vi "ExTestPutRowI32.vi"() -> ()   [LabVIEW 2010]
panel:
  out "Image Display 2":i32[][](graph)
  out "error out":errorcluster
  in  "error in (no error)":errorcluster
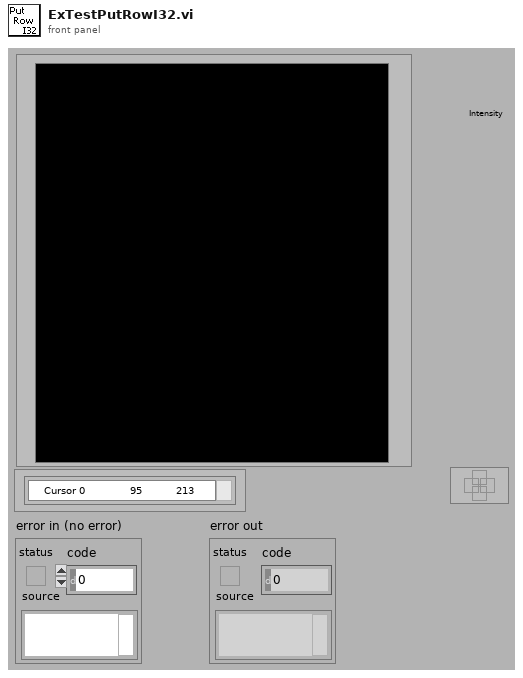
[diagram p1: front panel]
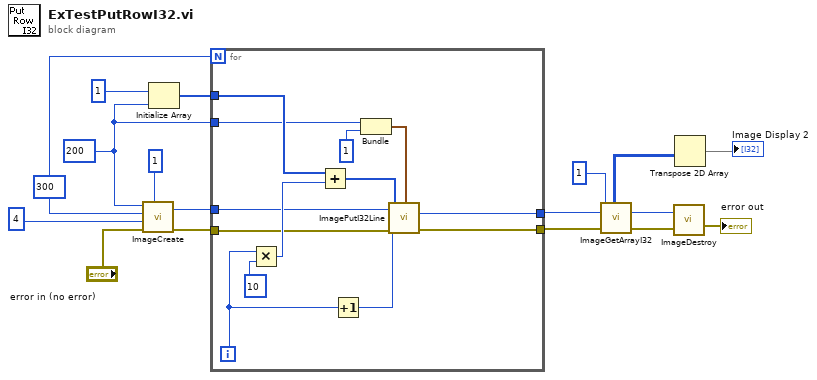
[diagram p0: block diagram]
diagram:
  w6 = 200
  w15 = 300
  n1 = call <userlib>:"ImageCreate.vi"("X dimension"=w6, "Y dimension"=w15, "Data Type"=4, "error in"="error in (no error)", "Number Of Frames"=1) -> ("Image Handle"=w7:u32, "error out"=w9:errorcluster)
  n2 = Initialize Array(1, w6) -> (w8:i32[])
  n3 = for {
    N: w15 -> [_]
    tunnel: w9 -> [w24]
    tunnel: w8 -> [w27]
    tunnel: w7 -> [w23]
    tunnel: w6 -> [w26]
    tunnel: [w21] -> w4
    tunnel: [w20] -> w3
    i -> [w30]
    n4 = Multiply(x=w30, y=10) -> (x*y=w28:i32)
    n5 = Add(x=w27, y=w28) -> (x+y=w18:i32[])
    n6 = Increment(x=w30) -> (x+1=w19:i32)
    n7 = Bundle(w26, 1) -> (w22:cluster{i32, i32})  [unwired: 1 in]
    n8 = call <userlib>:"ImagePutI32Line.vi"("Image Handle"=w23, "Image Data"=w18, "Y Position"=w19, "error in (no error)"=w24, "Image dimensions"=w22) -> ("Image Handle"=w20:u32, "error out"=w21:errorcluster)
  }
  n9 = call <userlib>:"ImageGetArrayI32.vi"("error in"=w4, "Z position"=1, "Image Handle"=w3) -> ("error out"=w5:errorcluster, "Array int 32"=w2:i32[][], "Image Handle"=w11:u32)
  n10 = call <userlib>:"ImageDestroy.vi"("error in"=w5, "Data handle"=w11) -> ("error out"=→"error out":errorcluster)
  n11 = Transpose 2D Array(2D array=w2) -> (transposed array=→"Image Display 2":i32[][])
